vi "RegisterAudioValidationServices.vi"   [LabVIEW 2021]
uses:
  <vilib>/Utility/sysdir.llb/System Directory Type.ctl
types:
  T1 = typedef "System Directory Type.ctl" = i32
  T2 = enum32{"Invalid", "Standard", "Closed", "Hidden", "Minimized", "Maximized"}
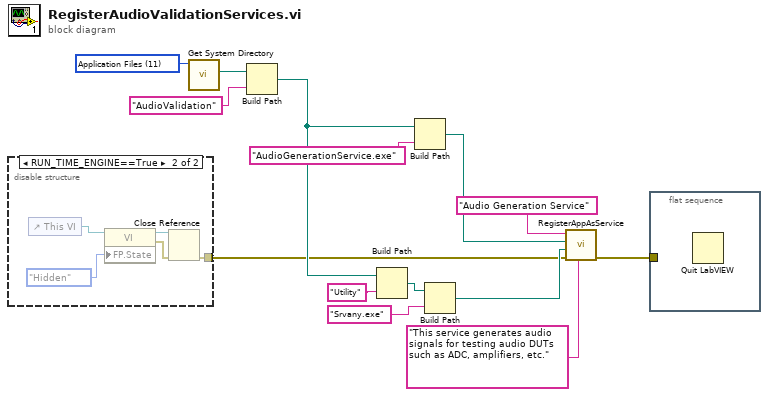
[diagram p0: block diagram]
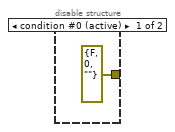
[diagram p2: hidden frame]
diagram:
  w14 = T1 11 items=["User Home"=0, "User Desktop"=1, "User Documents"=2, "User Application Data"=3, "User Preferences"=4, "User Temporary"=5, "Public Documents"=6, "Public Application Data"=7, "Public Preferences"=8, "Public Cache"=13, "System Core Libraries"=9, "System Installed Libraries"=10, "Application Files"=11, "Boot Volume Root"=12] ("system directory type")
  n1 = disable-structure shown="RUN_TIME_ENGINE==True" {
    disable-tunnel: [errorcluster {"status"=FALSE, "code"=0, "source"=""} ("error in (no error)") w16] -> w1
    frame condition #0 (active) {
    }
    frame condition #1 {
      n2 = control-ref of="This VI"() -> (w19:refnum<vi>)
      n3 = property class="VI"(reference=w19, "FP.State"=T2."Hidden" ("Front Panel Window:State")) -> (reference out=w18:refnum<vi>, error out=w17:errorcluster)  [unwired: 1 in]
      n4 = Close Reference(reference=w18, error in (no error)=w17) -> (error out=w16:errorcluster)
    }
  }
  n5 = call <vilib>:"Get System Directory.vi"("system directory type"=w14) -> ("system directory"=w13:path)  [unwired: 10 in]
  n6 = Build Path(base path=w13, name or relative path="AudioValidation") -> (appended path=w4:path)
  n7 = Build Path(base path=w4, name or relative path="Utility") -> (appended path=w9:path)
  n8 = Build Path(base path=w4, name or relative path="AudioGenerationService.exe") -> (appended path=w6:path)
  n9 = Build Path(base path=w9, name or relative path="Srvany.exe") -> (appended path=w5:path)
  n10 = call "RegisterAppAsService.vi"("service description"="This service generates audio signals for testing audio DUTs such as ADC, amplifiers, etc.", "error in (no error)"=w1, "SrvAny.exe Path"=w5, "app path"=w6, "service name"="Audio Generation Service") -> ("error out"=w2:errorcluster)  [unwired: 6 in]
  n11 = flat-sequence {
    tunnel: w2 -> [_]
    frame #0 {
      n12 = Quit LabVIEW() -> ()  [unwired: 1 in]
    }
  }
